vi "FaultState.vi"(8 "error in (no error)":errorcluster, 11 "CurrentState":T1) -> (0 "error out":errorcluster, 2 "Cluster":T2, 3 "CurrentState 2":T1)   [LabVIEW 2018]
uses:
  Type_Def/Type_Def Actuator Controls.ctl
  Type_Def/Type_Def ControlState.ctl
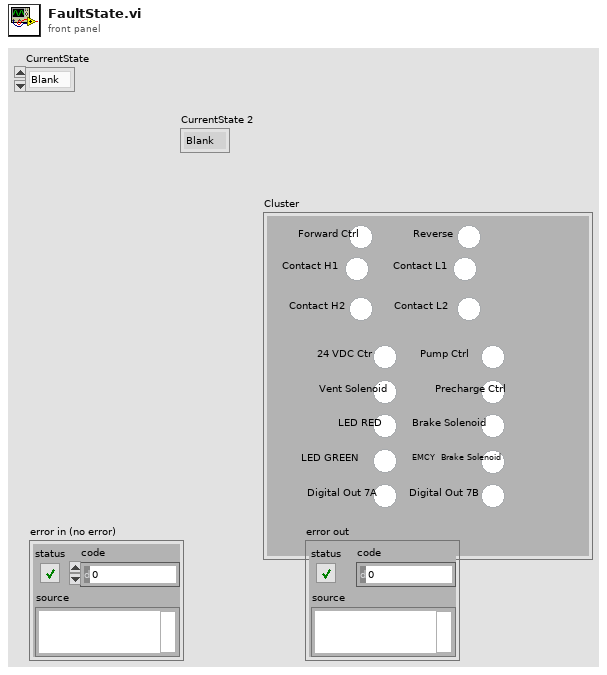
[diagram p1: front panel]
types:
  T1 = typedef "Type_Def ControlState.ctl" = enum16{"Blank", "Systems Check", "Idle", "Ready", "Pushing", "CrawlingPrecharge", "Braking", "Fault", "Boot Up", "Crawling", "Shutdown", "Service Push", "Service Wait", "Vent", "Precharge"}
  T2 = typedef "Type_Def Actuator Controls.ctl" = cluster{"Reverse ":bool, "Precharge Ctrl":bool, "Pump Ctrl":bool, "24 VDC Ctr":bool, "Vent Solenoid":bool, "Brake Solenoid":bool, "EMCY  Brake Solenoid":bool, "Digital Out 7B ":bool, "Forward Ctrl":bool, " Contact H2":bool, "Contact L2":bool, "LED RED":bool, "LED GREEN":bool, " Digital Out 7A":bool, " Contact H1":bool, "Contact L1":bool}
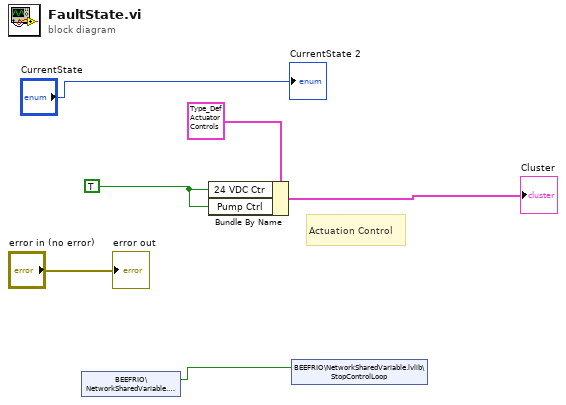
[diagram p0: block diagram]
diagram:
  w1 = TRUE
  # "Actuation Control"
  n1 = shared-variable "BEEFRIO\\NetworkSharedVariable.lvlib\\Shutdown"() -> (w3:bool)  [unwired: 1 in, 1 out]
  n2 = Bundle By Name(cluster=T2 {"Reverse "=FALSE, "Precharge Ctrl"=FALSE, "Pump Ctrl"=FALSE, "24 VDC Ctr"=FALSE, "Vent Solenoid"=FALSE, "Brake Solenoid"=FALSE, "EMCY  Brake Solenoid"=FALSE, "Digital Out 7B "=FALSE, "Forward Ctrl"=FALSE, " Contact H2"=FALSE, "Contact L2"=FALSE, "LED RED"=FALSE, "LED GREEN"=FALSE, " Digital Out 7A"=FALSE, " Contact H1"=FALSE, "Contact L1"=FALSE} ("Cluster in 2"), "24 VDC Ctr"=w1, "Pump Ctrl"=w1) -> (→"Cluster":T2)
  n3 = shared-variable "BEEFRIO\\NetworkSharedVariable.lvlib\\StopControlLoop"(w3) -> ()  [unwired: 1 in, 1 out]
  "error out" <- "error in (no error)"
  "CurrentState 2" <- "CurrentState"
